vi "Change Digits.vi"(8 "error in (no error)":errorcluster, 10 "Digits":i32, 11 "Numeric Data Type in":refnum<class "Numeric Data Type.lvclass">) -> (0 "error out":errorcluster, 3 "Numeric Data Type out":refnum<class "Numeric Data Type.lvclass">)   [LabVIEW 2018, in "Numeric Data Type.lvclass"]
uses:
  Numeric Data Type.lvclass
  Numeric Data Type.lvclass/Numeric Data Type.ctl
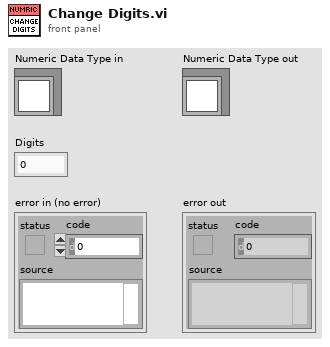
[diagram p1: front panel]
types:
  T1 = typedef "Numeric Data Type.lvclass/Numeric Info.ctl" = cluster{"Minimum Field Width":i32, "Digits of Precision":i32, "Numeric Format":T2, "Precision Type":T3, "Hide trailing zeros":bool, "exponent":bool, "just/pad":T4, "Modifiers":string}
  T2 = typedef "Numeric Data Type.lvclass/Numeric Format Enum.ctl" = enum16{"Floating Point Notation", "Scientific Notation", "Engineering Notation", "SI Notation", "<not used>", "Decimal", "Hexadecimal", "Octal", "Binary", "<not used 2>", "Absolute Time", "Relative Time"}
  T3 = typedef "Numeric Data Type.lvclass/Precision Type.ctl" = enum16{"Digits of precision", "Significant digits"}
  T4 = typedef "Numeric Data Type.lvclass/Padding.ctl" = enum16{"Pad with spaces on left", "Pad with spaces on right", "Pad with zeros on left"}
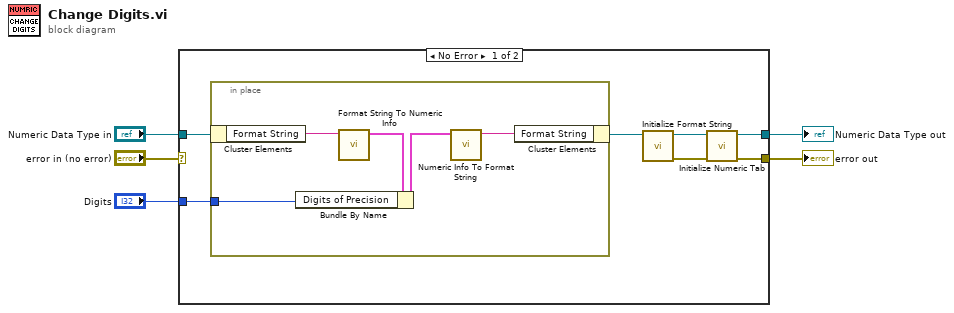
[diagram p0: block diagram]
diagram:
  n1 = case shown="No Error" "error in (no error)" {
    selector: "error in (no error)" -> [_ w19]
    tunnel: [w6 w19] -> w4
    tunnel: [w8 w18] -> w2
    tunnel: "Numeric Data Type in" -> [w12 w18]
    tunnel: "Digits" -> [w11 _]
    frame No Error {
      n2 = in-place {
        in-place-border: w11 -> [w15]
        n3 = in-place-cluster #1(w12) -> ("Format String"=w17:string)
        n4 = call "Format String To Numeric Info.vi"("Format String"=w17) -> ("Numeric Format & Precision Info"=w16:T1)  [unwired: 10 in]
        n5 = Bundle By Name(cluster=w16, "Digits of Precision"=w15) -> (w14:T1)
        n6 = call "Numeric Info To Format String.vi"("Numeric Format & Precision Info"=w14) -> ("Format String"=w13:string)  [unwired: 10 in]
        n7 = in-place-cluster #1("Format String"=w13) -> (w10:refnum<class "Numeric Data Type.lvclass">)
      }
      n8 = call "Initialize Format String.vi"("Numeric Data Type in"=w10) -> ("error out"=w7:errorcluster, "Numeric Data Type (dup)"=w9:refnum<class "Numeric Data Type.lvclass">)  [unwired: 9 in]
      n9 = call "Initialize Numeric Tab.vi"("error in (no error)"=w7, "Numeric Data Type in"=w9) -> ("error out"=w6:errorcluster, "Numeric Data Type (dub)"=w8:refnum<class "Numeric Data Type.lvclass">)  [unwired: 8 in]
    }
    frame Error {
    }
  }
  "error out" <- w4
  "Numeric Data Type out" <- w2
